vi "Spirometer Flow Integration.vi"(7 "Reset Integral":bool, 11 "Waveform in":waveform(dbl)) -> (3 "Waveform Array":waveform(dbl)[](array[waveform]))   [LabVIEW 2012]
uses:
  <vilib>/ptbypt/NI_PtbyPt.lvlib
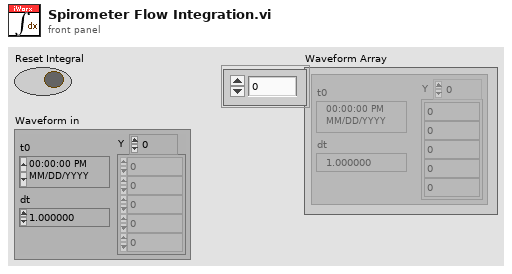
[diagram p1: front panel]
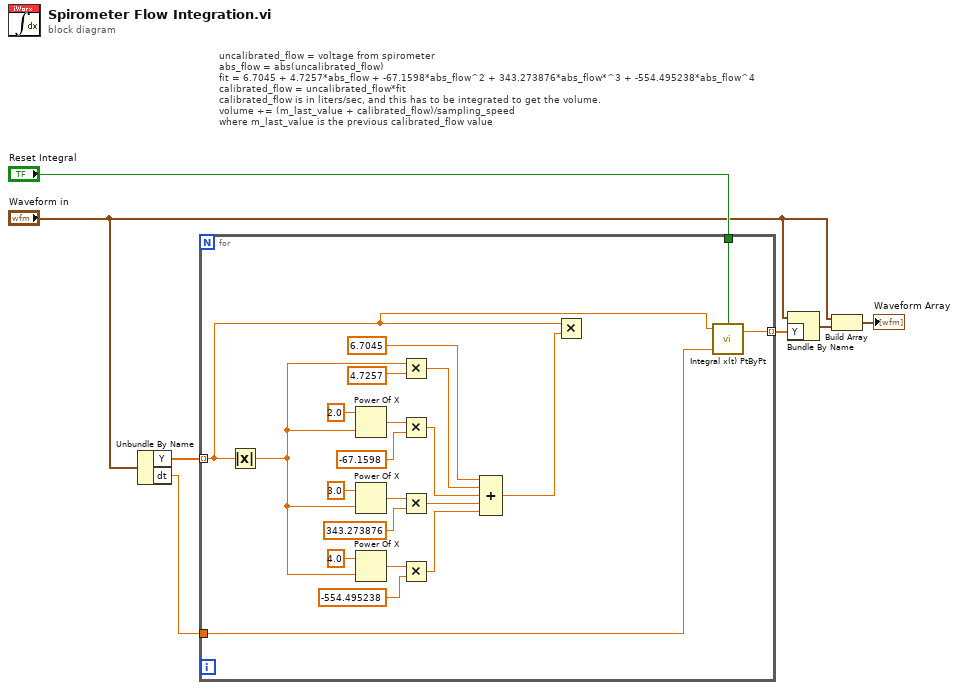
[diagram p0: block diagram]
diagram:
  # "uncalibrated_flow = voltage from spirometer\nabs_flow = abs(uncalibrated_flow)\nfit = 6.7045 + 4.7257*abs_flow + -67.1598*abs_flow^2 + 343.273876*abs_flow*^3 + -554.495238*abs_flow^4\ncalibrated_flow = uncalibrated_flow*fit\ncalibrated_flow is in liters/sec, and this has to be integrated to get the volume.\nvolume += (m_last_value + calibrated_flow)/sampling_speed\nwhere m_last_value is the previous calibrated_flow value"
  n1 = Unbundle By Name("Waveform in") -> ("Y"=w3:dbl[], "dt"=w1:dbl)
  n2 = for {
    tunnel: w3 -> [w8] mode=indexing
    tunnel: [w28] -> w4 mode=indexing
    tunnel: "Reset Integral" -> [w27]
    tunnel: w1 -> [w9]
    n3 = Absolute Value(x=w8) -> (abs(x)=w12:dbl)
    n4 = Power Of X(1:w12, 2:2.0 ("y")) -> (0:w21:dbl)
    n5 = Power Of X(1:w12, 2:3.0 ("y")) -> (0:w18:dbl)
    n6 = Power Of X(1:w12, 2:4.0 ("y")) -> (0:w14:dbl)
    n7 = Multiply(x=w12, y=4.7257 ("x")) -> (x*y=w24:dbl)
    n8 = Multiply(x=w21, y=-67.1598 ("x")) -> (x*y=w20:dbl)
    n9 = Multiply(x=w18, y=343.273876) -> (x*y=w16:dbl)
    n10 = Multiply(x=w14, y=-554.495238) -> (x*y=w11:dbl)
    n11 = Compound Arithmetic op=ADD(6.7045 ("x"), w24, w20, w16, w11) -> (w10:dbl)
    n12 = Multiply(x=w8, y=w10) -> ()  [unwired: 1 out]
    n13 = call <vilib>:"Integral x(t) PtByPt.vi"("initialize"=w27, "dt"=w9, "x"=w8) -> ("integral x(t)"=w28:dbl)  [unwired: 1 in, 1 out]
  }
  n14 = Bundle By Name(cluster="Waveform in", "Y"=w4) -> (w7:waveform(dbl))
  n15 = Build Array("Waveform in", w7) -> (→"Waveform Array":waveform(dbl)[])
